vi "Update All.vi"(0 "reference in":refnum<class "Temp.lvclass">, 5 "error in (no error)":errorcluster) -> (14 "reference out":refnum<class "Temp.lvclass">, 19 "error out":errorcluster)   [LabVIEW 2017, in "Temp.lvclass"]
uses:
  Temp.lvclass
  <vilib>/DAQmx/read.llb/DAQmx Read (Analog 1D DBL NChan 1Samp).vi
  <vilib>/DAQmx/miscellaneous.llb/DAQmx Fill In Error Info.vi
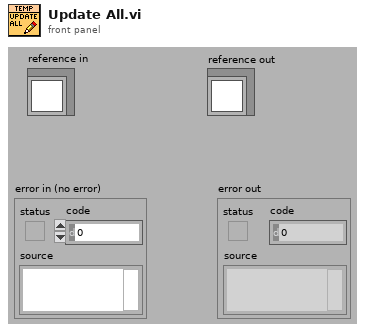
[diagram p1: front panel]
types:
  T1 = typedef "Temp.lvclass/ObjectAttributes.ctl" = cluster{"Temperature Task":refnum<k21>, "Temperature Readings":dbl[], "Thermocouple Type":i32, "Temperature Units":i32, "Average Temperature":dbl, "Number of Temperature Modules":i32, "Number of Total Temperature Channels":i32, "Temperature On/Off Status":bool, "Temperature Module Names (NI-Max Name)":string[], "Number of Channels Per Temperature  Module":i32[], "Temperature VI Reference":refnum<vi>}
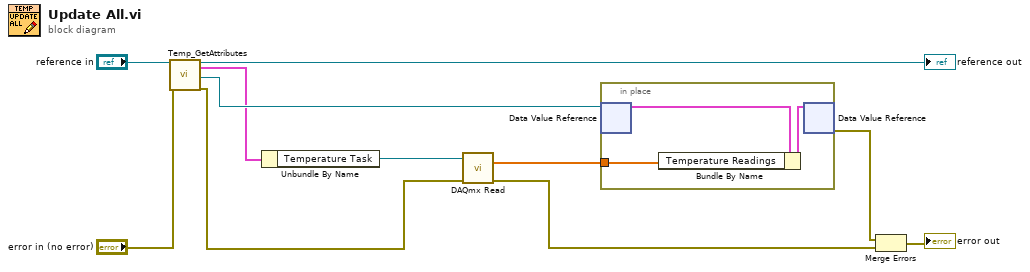
[diagram p0: block diagram]
diagram:
  n1 = call "Temp_GetAttributes.vi"("reference in"="reference in", "error in (no error)"="error in (no error)") -> ("reference out"=→"reference out":refnum<class "Temp.lvclass">, "Data"=w3:T1, "DataRef"=w6:refnum<data-value>, "error out"=w2:errorcluster)  [unwired: 14 in]
  n2 = Unbundle By Name(w3) -> ("Temperature Task"=w5:refnum<k21>)
  n3 = call-poly <vilib>:"DAQmx Read.vi"("task/channels in"=w5, "error in"=w2) -> ("data"=w4:dbl[], "error out"=w1:errorcluster)  [unwired: 11 in, 1 out]
  n4 = in-place {
    in-place-border: w4 -> [w12]
    n5 = in-place-dvr #1(w6) -> (w13:T1)  [unwired: 1 out]
    n6 = Bundle By Name(cluster=w13, "Temperature Readings"=w12) -> (w14:T1)
    n7 = in-place-dvr #1(w14) -> (w7:errorcluster)  [unwired: 1 out]
  }
  n8 = Merge Errors(w7, w1) -> (→"error out":errorcluster)
